vi "output check host.vi"() -> ()   [LabVIEW 2012]
uses:
  <vilib>/FPGAPlugInAG/cRIO-9082/niLvFpga_Open_cRIO-9082.vi
  <vilib>/rvi/interface/common/dynamic/niFpgaDynamicAddResources.vi
  <vilib>/Utility/error.llb/Error Cluster From Error Code.vi
  <vilib>/rvi/errors/niLvFpgaAdjustHostInterfaceError.vi
  <vilib>/FPGAPlugInAG/Dynamic/niLvFpga_Run_Dynamic.vi
  <vilib>/Utility/file.llb/Write To Spreadsheet File (I64).vi
  <vilib>/rvi/interface/nirviOpenFPGA/nirviOpenFPGA.xnode
  FPGA Bitfiles/simpletest_FPGATarget_outputcheckAI3_9rUv9DEy4Yk.lvbitx
  <vilib>/rvi/interface/nirviReadWriteControl/nirviReadWriteControl.xnode
  <vilib>/rvi/interface/nirviMethod/nirviMethod.xnode
  <vilib>/rvi/errors/niLvFpgaMergeErrorWithErrorCode.vi
  NiFpgaLv.dll
  <vilib>/rvi/interface/Simulation/niFpgaSimulationCallBeginRW.vi
  <vilib>/FPGAPlugInAG/Dynamic/niLvFpga_ConfigureFifo_Dynamic.vi
  <vilib>/FPGAPlugInAG/Dynamic/niLvFpga_StartFifo_Dynamic.vi
  <vilib>/FPGAPlugInAG/Dynamic/niLvFpga_ReadFifo_Dynamic.vi
panel:
  out "Elements Remaining":u32
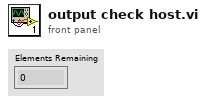
[diagram p1: front panel]
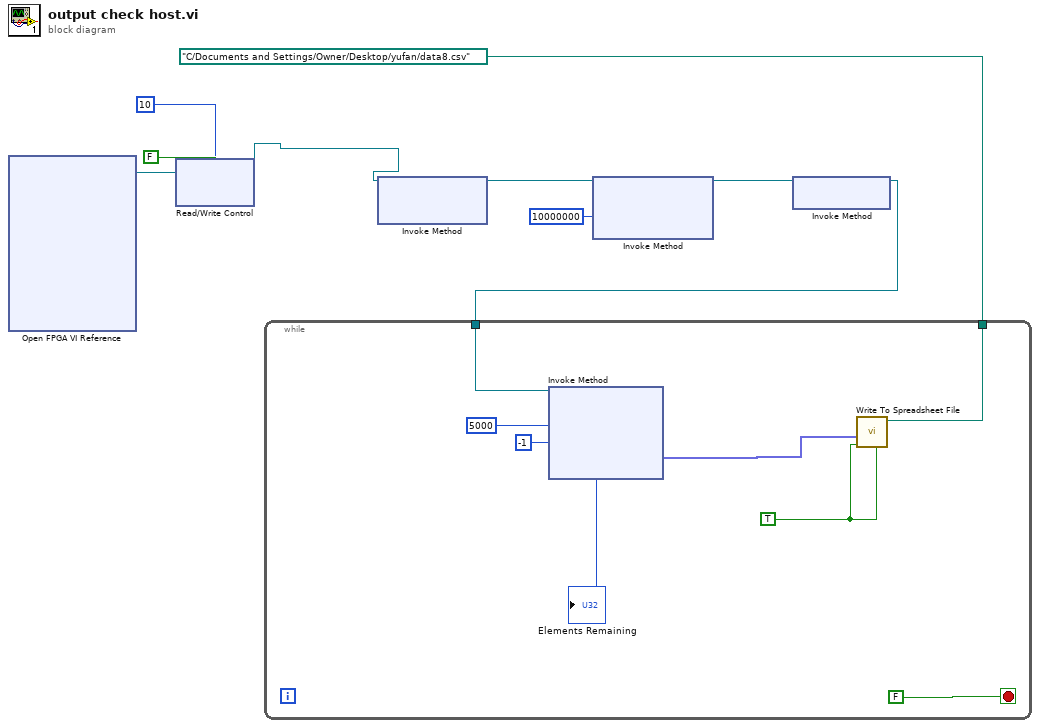
[diagram p0: block diagram]
diagram:
  n1 = xnode "Open FPGA VI Reference"() -> ("FPGA VI Reference Out"=w1:refnum<k20>)  [unwired: 2 in, 1 out]
  n2 = xnode "Read/Write Control"("FPGA VI Reference In"=w1, "stop"=FALSE, "Count(uSec)"=u32 10) -> ("FPGA VI Reference Out"=w4:refnum<k20>)  [unwired: 1 in, 1 out]
  n3 = xnode "Invoke Method"("FPGA VI Reference In"=w4) -> ("FPGA VI Reference Out"=w9:refnum<k20>)  [unwired: 2 in, 1 out]
  n4 = xnode "Invoke Method"("FPGA VI Reference In"=w9, "Requested Depth"=u32 10000000) -> ("FPGA VI Reference Out"=w7:refnum<k20>)  [unwired: 1 in, 2 out]
  n5 = xnode "Invoke Method"("FPGA VI Reference In"=w7) -> ("FPGA VI Reference Out"=w6:refnum<k20>)  [unwired: 1 in, 1 out]
  n6 = while {
    tunnel: w6 -> [w13]
    tunnel: path "C:/Documents and Settings/Owner/Desktop/yufan/data8.csv" ("file path (dialog if empty)") -> [w11]
    stop <- FALSE stop-if-true
    w15 = TRUE
    n7 = xnode "Invoke Method"("FPGA VI Reference In"=w13, "Number of Elements"=u32 5000, "Timeout (ms)"=-1) -> ("Data"=w14:fxp<+/-,32,32>[], "Elements Remaining"=→"Elements Remaining":u32)  [unwired: 1 in, 2 out]
    n8 = call-poly <vilib>:"Write To Spreadsheet File.vi"("transpose? (no:F)"=w15, "append to file? (new file:F)"=w15, "1D data"=w14, "file path (dialog if empty)"=w11) -> ()  [unwired: 4 in, 1 out]
  }
